vi "Relay Data Stream Control (Fast Side, Output).vi"(4 "ready for input?":bool=TRUE, 7 "state handshake":T1, 9 "data valid":bool=TRUE caption="data valid (true)", 10 "element count":u16=1 caption="element count (1)") -> (0 "permissed elements":u16, 1 "send data":bool, 2 "stream.state 0":T2, 3 "stream.samples transferred 0":u64, 6 "force data":bool)   [LabVIEW 2014, in "niInstr Streaming v1 FPGA.lvlib"]
uses:
  <instrlib>/_niInstr/Streaming/v1/FPGA/niInstr Streaming v1 FPGA.lvlib
  <instrlib>/_niInstr/Streaming/v1/Common/Stream State.ctl
  <instrlib>/_niInstr/Streaming/v1/FPGA/Public/Stream Additive Count Register.ctl
  <instrlib>/_niInstr/Streaming/v1/Common/niInstr Streaming v1 Common.lvlib
panel:
  in  "reset":bool caption="reset (optional)"
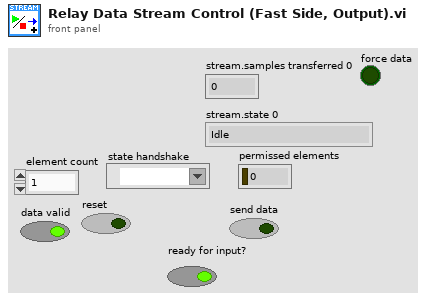
[diagram p1: front panel]
types:
  T1 = typedef "niInstr Streaming v1 FPGA.lvlib/Stream Additive Count Register.ctl" = refnum<k21>
  T2 = typedef "niInstr Streaming v1 Common.lvlib/Stream State.ctl" = enum8{"Idle", "Finite Transfer", "Continuous", "Done", "Overflow", "Not Ready", "Cancel"}
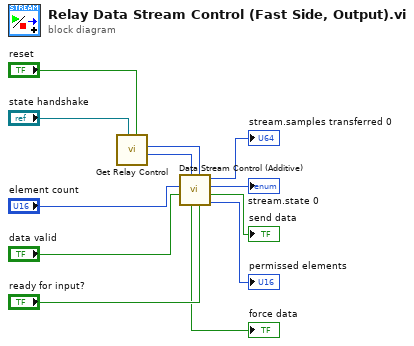
[diagram p0: block diagram]
diagram:
  n1 = call <instrlib>:"Get Relay Control.vi"("reset"="reset", "state handshake"="state handshake") -> ("stream.state n"=w11:T2, "additive num samples"=w12:u16)  [unwired: 8 in]
  n2 = call <instrlib>:"Data Stream Control (Additive).vi"("ready for input?"="ready for input?", "stream.additive num samples 0"=w12, "stream.request state 0"=w11, "data valid"="data valid", "element count"="element count") -> ("permissed elements"=→"permissed elements":u16, "send data"=→"send data":bool, "stream.state 0"=→"stream.state 0":T2, "stream.samples transferred 0"=→"stream.samples transferred 0":u64, "force data"=→"force data":bool)  [unwired: 2 in]
